vi "Autonomous Independent.vi"   [LabVIEW 2013]
doc: "This VI is called when autonomous begins, and will automatically be terminated when autonomous ends. You can carry out timed or sensor driven robot movement independently without needing to return to the caller."
uses:
  Robot Global Data.vi
  Gyro/Gyro Global.vi
types:
  T1 = typedef "WPI_GyroDevRef.ctl" = cluster{"DevStatus":errorcluster, "Analog Module":T2, "Analog Channel":T3, "Offset":dbl, "Gain (VoltsPerDegree/Second)":dbl}
  T2 = typedef "FPGA_TypedefAnalogModule.ctl" = enum16{"Analog Module 1", "Analog Module 2"}
  T3 = typedef "FPGA_AIChannel.ctl" = enum8{"AI 1", "AI 2", "AI 3", "AI 4", "AI 5", "AI 6", "AI 7", "AI 8", "Invalid"}
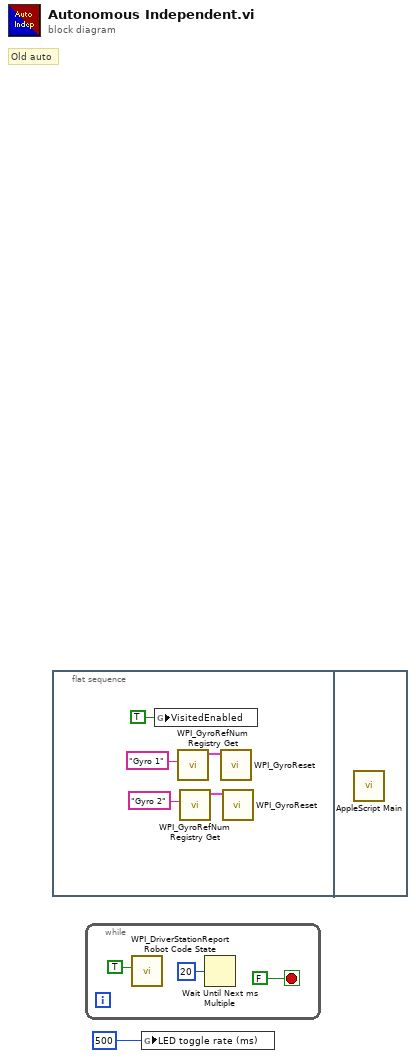
[diagram p0: block diagram]
diagram:
  # "Old auto"
  n1 = flat-sequence {
    frame #0 {
      n2 = global write "Gyro Global.vi" "VisitedEnabled"(TRUE ("VisitedEnabled")) -> ()
      n3 = call <vilib>:"WPI_GyroRefNum Registry Get.vi"("refnum name"="Gyro 1") -> ("GyroDevRef"=w5:T1)  [unwired: 9 in, 1 out]
      n4 = call <vilib>:"WPI_GyroRefNum Registry Get.vi"("refnum name"="Gyro 2") -> ("GyroDevRef"=w4:T1)  [unwired: 9 in, 1 out]
      n5 = call <vilib>:"WPI_GyroReset.vi"("GyroDevRef"=w5) -> ()  [unwired: 9 in, 2 out]
      n6 = call <vilib>:"WPI_GyroReset.vi"("GyroDevRef"=w4) -> ()  [unwired: 9 in, 2 out]
    }
    frame #1 {
      n7 = call "AppleScript Main.vi"() -> ()  [unwired: 12 in]
    }
  }
  n8 = while {
    stop <- FALSE stop-if-true
    n9 = call <vilib>:"WPI_DriverStationReport Robot Code State.vi"("Autonomous"=TRUE) -> ()  [unwired: 10 in, 1 out]
    n10 = Wait Until Next ms Multiple(millisecond multiple=u32 20 ("milliseconds to wait")) -> ()  [unwired: 1 out]
  }
  n11 = global write "Robot Global Data.vi" "LED toggle rate (ms)"(u32 500 ("LED ms toggle rate")) -> ()
